vi "Unflatten.vi"(8 "error in (no error)":errorcluster, 11 "Voltage Pulse Gating System (HV supply) in":refnum<class "Voltage Pulse Gating System (HV supply).lvclass">) -> (0 "error out":errorcluster, 3 "Voltage Pulse Gating System (HV supply) out":refnum<class "Voltage Pulse Gating System (HV supply).lvclass">)   [LabVIEW 2017, in "Voltage Pulse Gating System (HV supply).lvclass"]
uses:
  Voltage Pulse Gating System (HV supply).lvclass
  Scanner/Scanner.lvclass
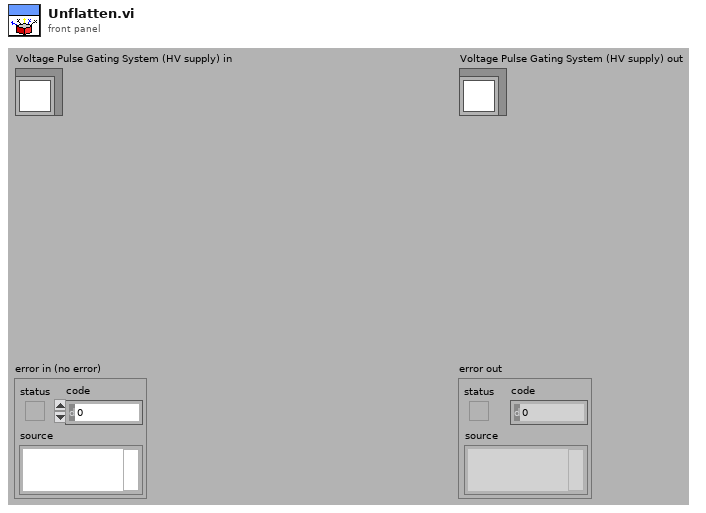
[diagram p1: front panel]
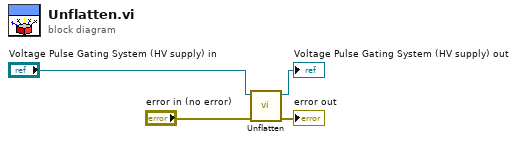
[diagram p0: block diagram]
diagram:
  n1 = call-parent "Unflatten.vi"("error in (no error)"="error in (no error)", "Scanner in"="Voltage Pulse Gating System (HV supply) in") -> ("error out"=→"error out":errorcluster, "Scanner out"=→"Voltage Pulse Gating System (HV supply) out":refnum<class "Voltage Pulse Gating System (HV supply).lvclass">)  [unwired: 8 in]
